vi "ALP4 B.vi"() -> ()   [LabVIEW 2016]
doc: "This Vi is a simple 4 way intersection street where the program has 3 modes, automatic, blink, all on test. The default is the automatic where it transist to simulate how a real life 4 way intersection works. The user is able to choose between those 3 states, the blink state just make it blink and the all on test makes everything to light up.\n\nAlexis Lopez\nP350\nCSUSB Physics"
uses:
  typedefs/stop light.ctl
  typedefs/left arrow.ctl
  typedefs/walk light.ctl
  typedefs/control mode enum.ctl
  typedefs/system state cluster.ctl
  typedefs/state enum.ctl
panel:
  out "system state":T1
  in  "mode set":T3
  in  "exit":bool
  out "WS walk":T4
  out "WN walk":T4
  out "ES walk":T4
  out "EN walk":T4
  out "SE walk":T4=TRUE
  out "SW walk":T4=TRUE
  out "NE walk":T4=TRUE
  out "NW walk":T4=TRUE
  out "East Light":T5={"stop"=FALSE, "caution"=FALSE, "go"=TRUE, "arrow"=FALSE}
  out "West Light":T5={"stop"=FALSE, "caution"=FALSE, "go"=TRUE, "arrow"=FALSE}
  out "North Light":T5={"stop"=TRUE, "caution"=FALSE, "go"=FALSE, "arrow"=FALSE}
  out "South Light":T5={"stop"=TRUE, "caution"=FALSE, "go"=FALSE, "arrow"=FALSE}
  # "Alexis Lopez\nP350\nCSUSB Physics"
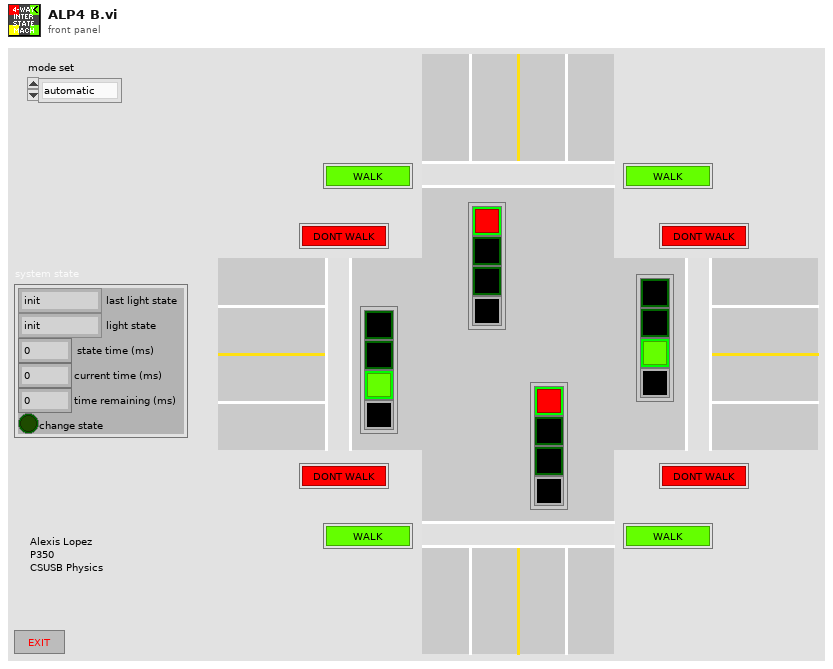
[diagram p1: front panel]
types:
  T1 = typedef "system state cluster.ctl" = cluster{"last light state":T2, "light state":T2, "state time (ms)":i32, "current time (ms)":i32, "time remaining (ms)":i32, "change state":bool}
  T2 = typedef "state enum.ctl" = enum16{"init", "idle", "left turn E", "go EW", "caution EW", "left turn W", "left turn N", "go NS", "caution NS", "left turn S", "blink on", "blink off", "all on test", "exit"}
  T3 = typedef "control mode enum.ctl" = enum16{"automatic", "blinking", "all on test"}
  T4 = typedef "walk light.ctl" = bool
  T5 = typedef "stop light.ctl" = cluster{"stop":bool, "caution":bool, "go":bool, "arrow":T6}
  T6 = typedef "left arrow.ctl" = bool
  T7 = typedef "all lights.ctl" = cluster{"east lights":T8, "west lights":T8, "north lights":T8, "south lights":T8}
  T8 = typedef "light set.ctl" = cluster{"light":T5, "walk A":T4, "walk B":T4}
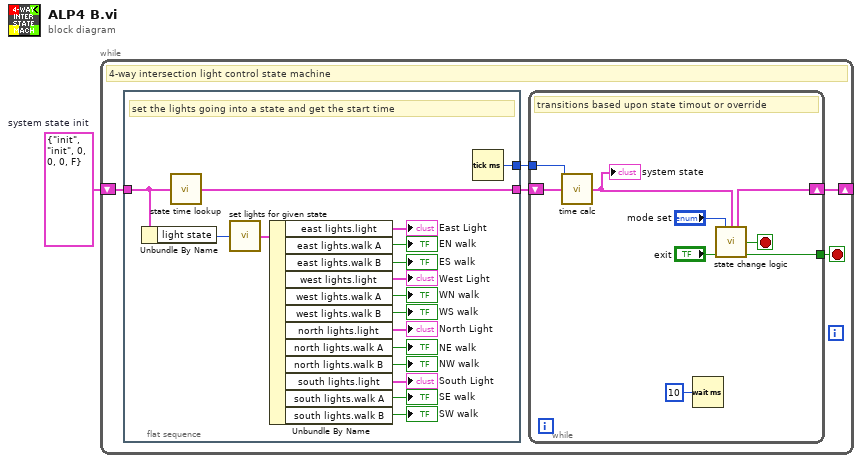
[diagram p0: block diagram]
diagram:
  w1 = T1 {"last light state"=enum."init", "light state"=enum."init", "state time (ms)"=0, "current time (ms)"=0, "time remaining (ms)"=0, "change state"=FALSE}  # system state init
  n1 = while {
    shift-right: [w4] -> _
    shift-left: w1 -> [w6]
    stop <- w3 stop-if-true
    # "4-way intersection light control state machine"
    n2 = flat-sequence {
      tunnel: w6 -> [w32]
      tunnel: [w17] -> w5
      tunnel: [w16] -> w2
      frame #0 {
        # "set the lights going into a state and get the start time"
        n3 = Unbundle By Name(w32) -> ("light state"=w18:T2)
        n4 = call "state time lookup.vi"("system state in"=w32) -> ("system state out"=w17:T1)  [unwired: 14 in]
        n5 = call "set lights for given state.vi"("light state"=w18) -> ("all lights out"=w31:T7)  [unwired: 14 in]
        n6 = Unbundle By Name(w31) -> ("east lights.light"=→"East Light":T5, "east lights.walk A"=→"EN walk":T4, "east lights.walk B"=→"ES walk":T4, "west lights.light"=→"West Light":T5, "west lights.walk A"=→"WN walk":T4, "west lights.walk B"=→"WS walk":T4, "north lights.light"=→"North Light":T5, "north lights.walk A"=→"NE walk":T4, "north lights.walk B"=→"NW walk":T4, "south lights.light"=→"South Light":T5, "south lights.walk A"=→"SE walk":T4, "south lights.walk B"=→"SW walk":T4)
        n7 = Tick Count (ms)() -> (millisecond timer value=w16:u32)
      }
    }
    n8 = while {
      shift-right: [w13] -> w4
      shift-left: w5 -> [w9]
      tunnel: [w12] -> w3
      tunnel: w2 -> [w8]
      stop <- w15 stop-if-true
      # "transitions based upon state timout or override"
      n9 = call "time calc.vi"("millisecond timer value"=w8, "system state in"=w9) -> ("system state out"=w7:T1)  [unwired: 13 in]
      "system state" <- w7
      n10 = Wait (ms)(milliseconds to wait=u32 10) -> ()  [unwired: 1 out]
      n11 = call "state change logic.vi"("mode set"="mode set", "system state in"=w7, "exit"="exit") -> ("system state out"=w13:T1, "change state"=w15:bool, "exit program"=w12:bool)  [unwired: 10 in]
    }
  }
